vi "ModifyClassAttribute2.vi"(5 "error in (no error)":errorcluster) -> (19 "error out":errorcluster)   [LabVIEW 2010, in "G#SubSubClass2.lvclass"]
uses:
  G#SubSubClass2.lvclass
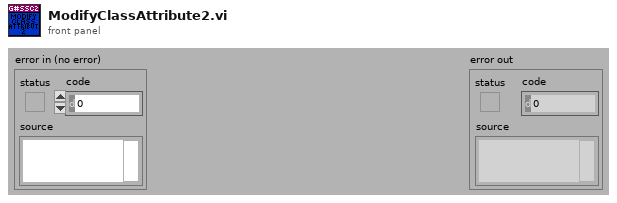
[diagram p1: front panel]
types:
  T1 = typedef "G#SubSubClass2.lvclass/ClassAttributes.ctl" = cluster{"Base class":T2, "SubSubClassAttr":i32}
  T2 = typedef "G#SubClass2.lvclass/ClassAttributes.ctl" = cluster{"Base class":T3, "SubClassAttr":i32}
  T3 = typedef "G#BaseClass2.lvclass/ClassAttributes.ctl" = cluster{"ClassAttr":i32}
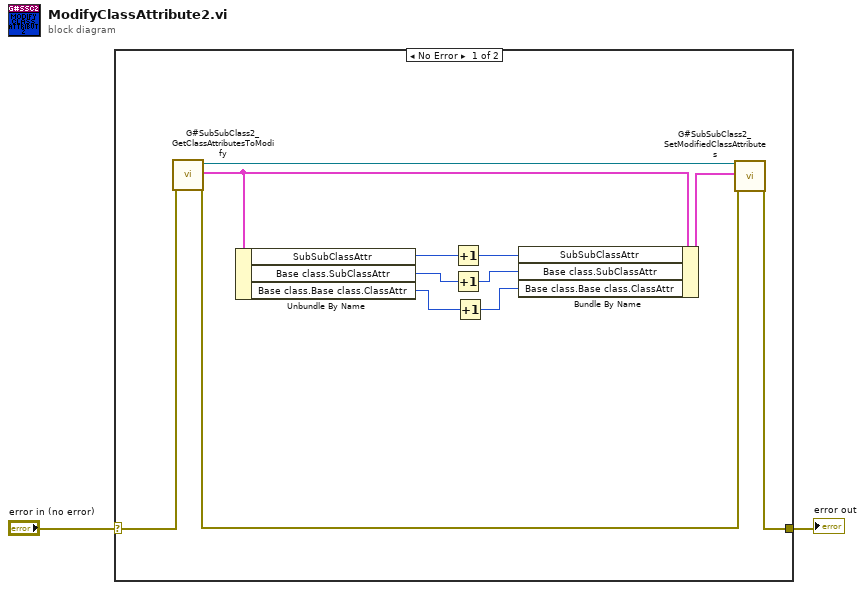
[diagram p0: block diagram]
diagram:
  n1 = case shown="No Error" "error in (no error)" {
    selector: "error in (no error)" -> [w10 w15]
    tunnel: [w12 w15] -> w1
    frame No Error {
      n2 = call "G#SubSubClass2_GetClassAttributesToModify.vi"("error in (no error)"=w10) -> ("reference out"=w13:refnum<class "G#SubSubClass2.lvclass">, "class attributes"=w9:T1, "error out"=w11:errorcluster)  [unwired: 13 in, 3 out]
      n3 = Unbundle By Name(w9) -> ("SubSubClassAttr"=w8:i32, "Base class.SubClassAttr"=w6:i32, "Base class.Base class.ClassAttr"=w4:i32)
      n4 = Increment(x=w8) -> (x+1=w7:i32)
      n5 = Increment(x=w6) -> (x+1=w5:i32)
      n6 = Increment(x=w4) -> (x+1=w3:i32)
      n7 = Bundle By Name(cluster=w9, "SubSubClassAttr"=w7, "Base class.SubClassAttr"=w5, "Base class.Base class.ClassAttr"=w3) -> (w14:T1)
      n8 = call "G#SubSubClass2_SetModifiedClassAttributes.vi"("reference in"=w13, "attributes"=w14, "error in (no error)"=w11) -> ("error out"=w12:errorcluster)  [unwired: 15 in, 1 out]
    }
    frame Error {
    }
  }
  "error out" <- w1
